vi "Change in Product Installers.vi"(8 "error in (no error)":errorcluster, 10 "Product Installers":T1[](array[typedef]), 11 "Bundle Builder in":refnum<class "Bundle Builder.lvclass">) -> (0 "error out":errorcluster, 1 "Custom Actions File Names":string[](array[string]), 2 "Product List File Names":string[](array[string]), 3 "Bundle Builder out":refnum<class "Bundle Builder.lvclass">, 4 "Bundle Filename":string)   [LabVIEW 2020, in "Bundle Builder.lvclass"]
uses:
  Bundle Builder.lvclass
  Typedef/Product Installer.ctl
  Bundle Builder.lvclass/Bundle Builder.ctl
  Typedef/Product Installer Definition.ctl
  4f63f28f-5265-4602-8317-7e5f909f2807.vi
  5d65ce95-3f27-4ad9-b4d3-753b2ea8e44f.vi
  <vilib>/Comparison/Equal/Equal Functor/Equal Functor.lvclass
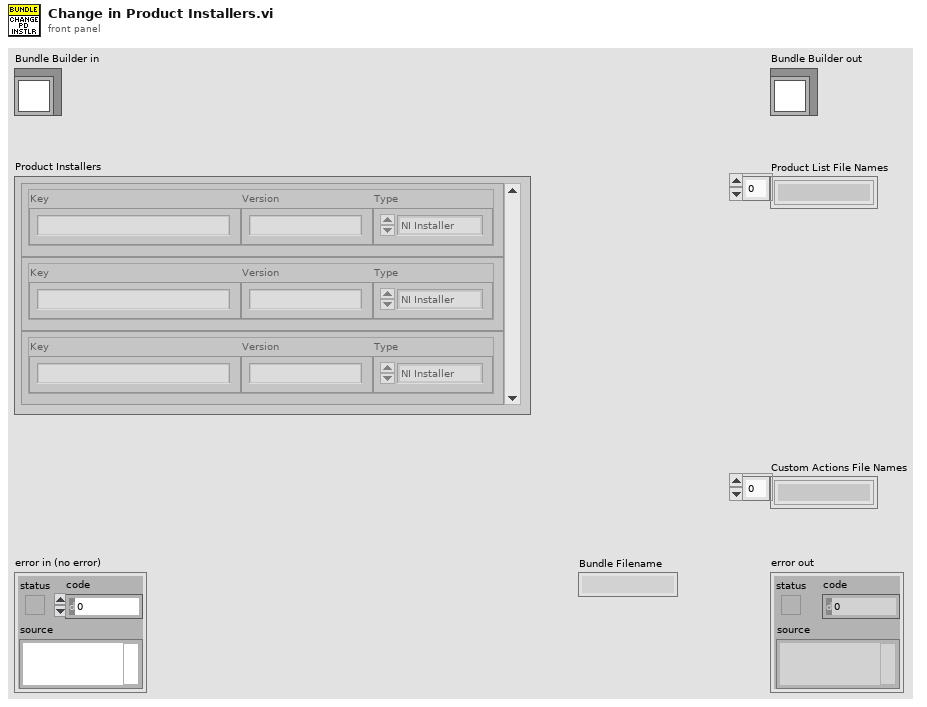
[diagram p1: front panel]
types:
  T1 = typedef "Product Installer.ctl" = cluster{"Key":string, "Version":string, "Type":enum16{"NI Installer", "Custom Installer"}}
  T2 = enum16{"All Elements Deleted", "Element Deleted", "Element Inserted", "Element Content Changed"}
  T3 = typedef "Product Installer Definition.ctl" = cluster{"Display Name":string, "Install Commands":cluster{"Path":string, "Parameters":string, "Successful Exit Codes":string, "Log Command":cluster{"Flag":string, "File Name":string}}[], "Uninstall Commands":cluster{"Path":string, "Parameters":string, "Successful Exit Codes":string, "Log Command":cluster{"Flag":string, "File Name":string}}[]}
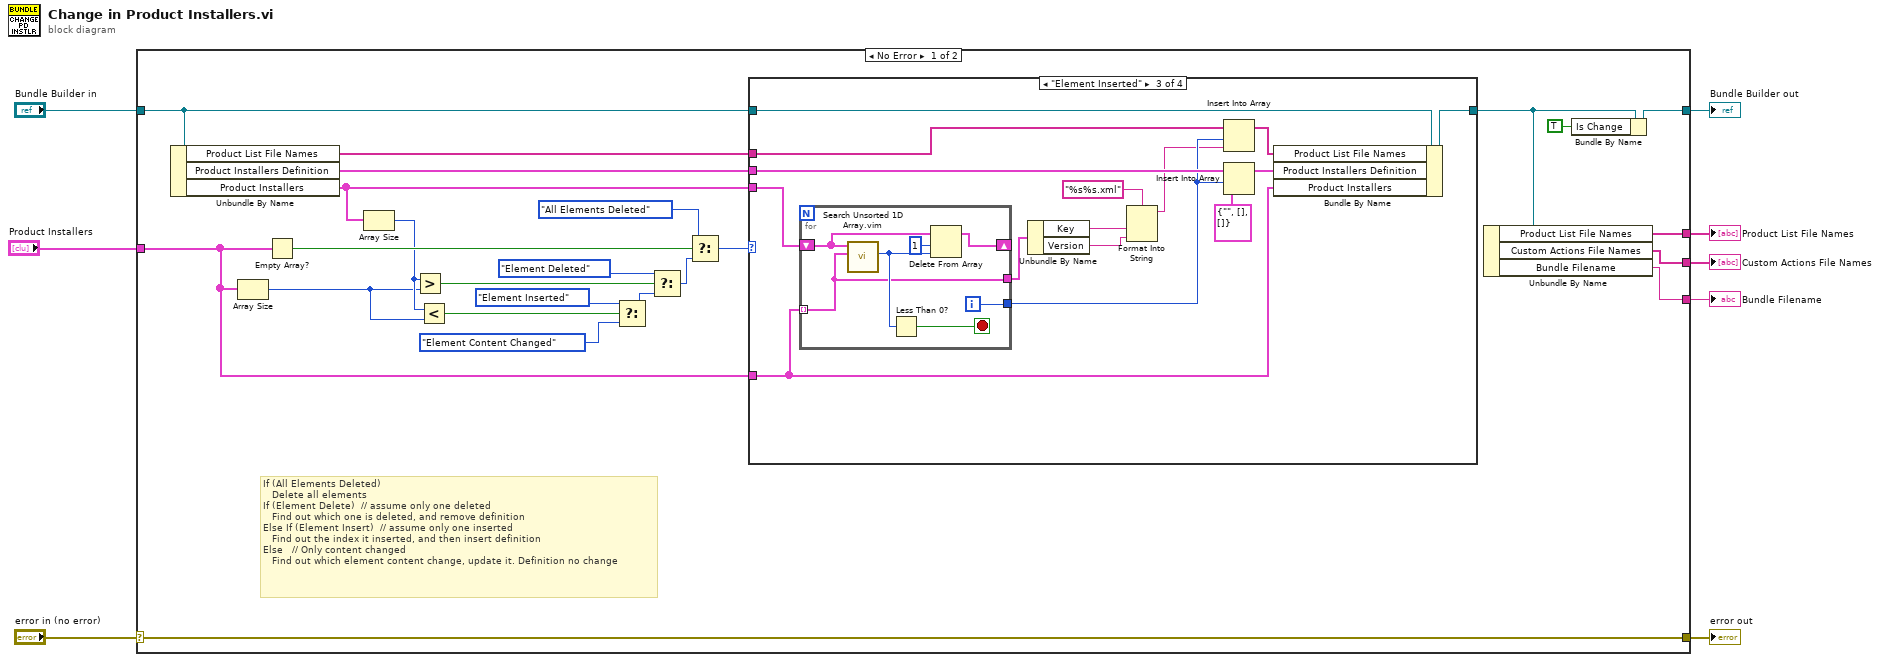
[diagram p0: block diagram]
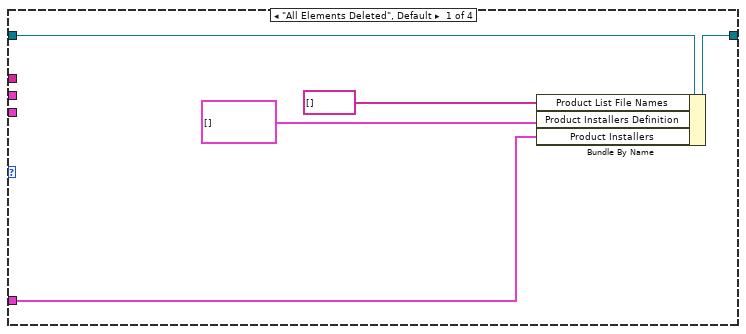
[diagram p2: hidden frame]
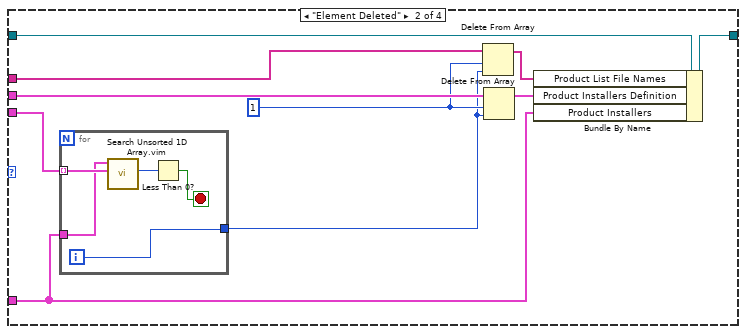
[diagram p3: hidden frame]
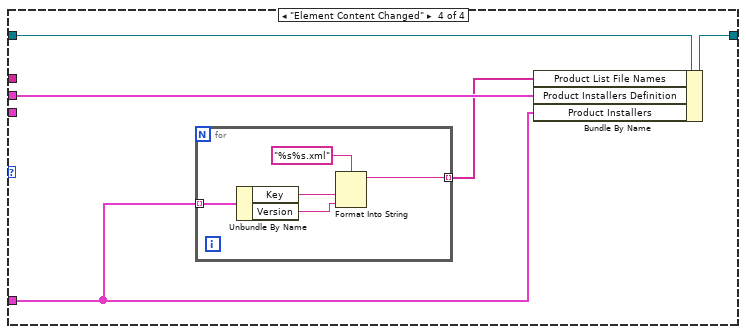
[diagram p4: hidden frame]
diagram:
  n1 = case shown="No Error" "error in (no error)" {
    selector: "error in (no error)" -> [w32 w86]
    tunnel: [w32 w86] -> w7
    tunnel: [w10 w85] -> w5
    tunnel: "Bundle Builder in" -> [w19 w85]
    tunnel: "Product Installers" -> [w18 _]
    tunnel: [w13 _] -> w3
    tunnel: [w12 _] -> w2
    tunnel: [w11 _] -> w1
    frame No Error {
      # "If (All Elements Deleted)\n   Delete all elements\nIf (Element Delete)  // assume only one deleted\n   Find out which one is deleted, and remove definition\nElse If (Element Insert)  // assume only one inserted\n   Find out the index it inserted, and then insert definition\nElse   // Only content changed\n   Find out which element content change, update it. Definition no change"
      n2 = Unbundle By Name(w19) -> ("Product List File Names"=w14:string[], "Product Installers Definition"=w16:T3[], "Product Installers"=w17:T1[])
      n3 = Array Size(array=w18) -> (size(s)=w25:i32)
      n4 = Empty Array?(array=w18) -> (empty?=w31:bool)
      n5 = Array Size(array=w17) -> (size(s)=w26:i32)
      n6 = Greater?(x=w26, y=w25) -> (0:w27:bool)
      n7 = Less?(x=w26, y=w25) -> (x < y?=w22:bool)
      n8 = Select(t=T2."Element Inserted", s=w22, f=T2."Element Content Changed") -> (s? t:f=w24:T2)
      n9 = Select(t=T2."Element Deleted", s=w27, f=w24) -> (s? t:f=w28:T2)
      n10 = Select(t=T2."All Elements Deleted", s=w31, f=w28) -> (s? t:f=w20:T2)
      n11 = case shown="\"Element Inserted\"" w20 {
        tunnel: w19 -> [w37 w47 w67 w79]
        tunnel: [w36 w46 w66 w78] -> w15
        tunnel: w18 -> [w34 w42 w61 w76]
        tunnel: w17 -> [_ w45 w65 _]
        tunnel: w16 -> [_ w44 w64 w77]
        tunnel: w14 -> [_ w41 w60 _]
        frame "All Elements Deleted", Default {
          n12 = Bundle By Name(cluster=w37, "Product List File Names"=string[] [], "Product Installers Definition"=T3[] [], "Product Installers"=w34) -> (w36:refnum<class "Bundle Builder.lvclass">)
        }
        frame "Element Deleted" {
          w39 = 1 ("length")
          n13 = for {
            tunnel: w45 -> [w52] mode=indexing
            tunnel: w42 -> [w51]
            tunnel: [w48] -> w38
            i -> [w48]
            stop <- w50 stop-if-true
            n14 = call "Search Unsorted 1D Array.vim"("element"=w52, "unsorted 1D array"=w51) -> ("index of element"=w49:i32)  [unwired: 9 in]
            n15 = Less Than 0?(x=w49) -> (x < 0?=w50:bool)
          }
          n16 = Delete From Array(array=w41, length=w39, index=w38) -> (array with subset deleted=w40:string[])  [unwired: 1 out]
          n17 = Delete From Array(array=w44, length=w39, index=w38) -> (array with subset deleted=w43:T3[])  [unwired: 1 out]
          n18 = Bundle By Name(cluster=w47, "Product List File Names"=w40, "Product Installers Definition"=w43, "Product Installers"=w42) -> (w46:refnum<class "Bundle Builder.lvclass">)
        }
        frame "Element Inserted" {
          n19 = for {
            tunnel: w61 -> [w68] mode=indexing
            tunnel: [w73] -> w59
            shift-right: [w69] -> _
            shift-left: w65 -> [w72]
            tunnel: [w68] -> w58
            i -> [w73]
            stop <- w74 stop-if-true
            n20 = call "Search Unsorted 1D Array.vim"("element"=w68, "unsorted 1D array"=w72) -> ("index of element"=w71:i32)  [unwired: 9 in]
            n21 = Less Than 0?(x=w71) -> (x < 0?=w74:bool)
            n22 = Delete From Array(array=w72, length=1, index=w71) -> (array with subset deleted=w69:T1[])  [unwired: 1 out]
          }
          n23 = Unbundle By Name(w58) -> ("Key"=w56:string, "Version"=w55:string)
          n24 = Format Into String(format string="%s%s.xml", w56, w55) -> (resulting string=w54:string)  [unwired: 2 in, 1 out]
          n25 = Insert Into Array(array=w60, index=w59, new element=w54) -> (w53:string[])
          n26 = Insert Into Array(array=w64, index=w59, new element=T3 {"Display Name"="", "Install Commands"=[], "Uninstall Commands"=[]} ("new element/subarray")) -> (w63:T3[])
          n27 = Bundle By Name(cluster=w67, "Product List File Names"=w53, "Product Installers Definition"=w63, "Product Installers"=w61) -> (w66:refnum<class "Bundle Builder.lvclass">)
        }
        frame "Element Content Changed" {
          n28 = for {
            tunnel: w76 -> [w81] mode=indexing
            tunnel: [w80] -> w75 mode=indexing
            n29 = Unbundle By Name(w81) -> ("Key"=w83:string, "Version"=w82:string)
            n30 = Format Into String(format string="%s%s.xml", w83, w82) -> (resulting string=w80:string)  [unwired: 2 in, 1 out]
          }
          n31 = Bundle By Name(cluster=w79, "Product List File Names"=w75, "Product Installers Definition"=w77, "Product Installers"=w76) -> (w78:refnum<class "Bundle Builder.lvclass">)
        }
      }
      n32 = Unbundle By Name(w15) -> ("Product List File Names"=w13:string[], "Custom Actions File Names"=w12:string[], "Bundle Filename"=w11:string)
      n33 = Bundle By Name(cluster=w15, "Is Change"=TRUE) -> (w10:refnum<class "Bundle Builder.lvclass">)
    }
    frame Error {
    }
  }
  "error out" <- w7
  "Bundle Builder out" <- w5
  "Product List File Names" <- w3
  "Custom Actions File Names" <- w2
  "Bundle Filename" <- w1
